vi "NET_Cube_Steer.vi"(8 "Read(F) Write(T)":bool, 9 "Max Speed In":dbl, 10 "Deadband In":dbl, 11 "Scale In":dbl) -> (1 "Max Speed Out":dbl, 2 "Deadband Out":dbl, 3 "Scale Out":dbl)   [LabVIEW 2017]
uses:
  <vilib>/Rock Robotics/Network Tables/NT Read Numeric Array.vi
  <vilib>/Rock Robotics/Network Tables/NT Write Numeric Array.vi
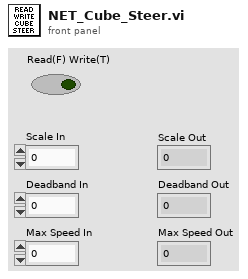
[diagram p1: front panel]
types:
  T1 = cluster{"Scale In":dbl, "Deadband In":dbl, "Max Speed In":dbl}
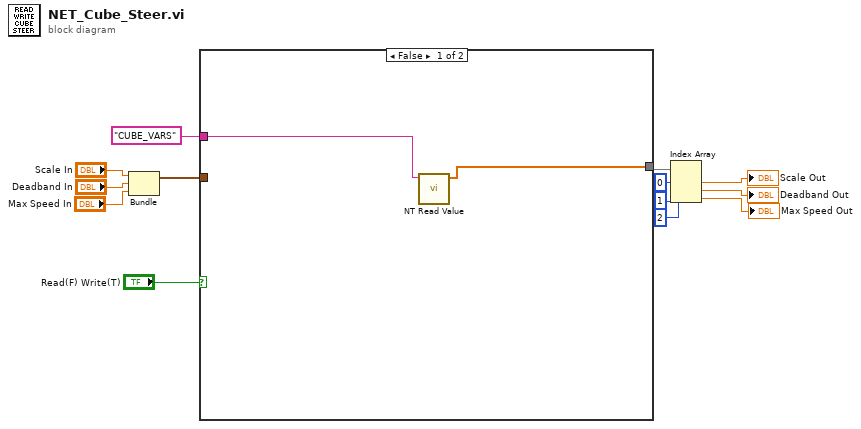
[diagram p0: block diagram]
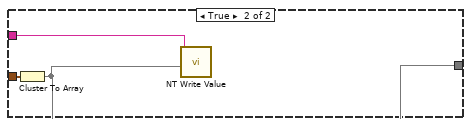
[diagram p2: hidden frame]
diagram:
  n1 = Bundle("Scale In"="Scale In", "Deadband In"="Deadband In", "Max Speed In"="Max Speed In") -> (w9:T1)  [unwired: 1 in]
  n2 = case shown="False" "Read(F) Write(T)" {
    tunnel: "CUBE_VARS" ("Name") -> [w15 w18]
    tunnel: [w14 w16] -> w8
    tunnel: w9 -> [_ w17]
    frame False {
      n3 = call-poly <vilib>:"NT Read Value.vi"("Name"=w15) -> ("Numeric Array"=w14:dbl[])  [unwired: 9 in, 1 out]
    }
    frame True {
      n4 = Cluster To Array(cluster=w17) -> (array=w16:dbl[])
      n5 = call-poly <vilib>:"NT Write Value.vi"("Numeric Array"=w16, "Name"=w18) -> ()  [unwired: 9 in, 1 out]
    }
  }
  n6 = Index Array(array=w8, index #1=0 ("index"), index #2=1 ("index"), index #3=2 ("index")) -> (element #1=→"Scale Out":dbl, element #2=→"Deadband Out":dbl, element #3=→"Max Speed Out":dbl)
